vi "CLASS - Generate2DTest.vi"(8 "error in (no error)":errorcluster, 11 "Local":T6) -> (0 "error out":errorcluster, 3 "Local Out":T6)   [LabVIEW 2020]
doc: "Generate the 2D graph"
uses:
  Controls/2DParameters.ctl
  _Controls/Datas.ctl
  _Controls/PointPropertyMultipleLabel.ctl
  _Controls/Style.ctl
  _Controls/2DData.ctl
types:
  T1 = typedef "2DParameters.ctl" = cluster{"Plot":refnum<vi>, "Data":T2, "Display":cluster{"Choice":enum16{"All", "Train", "Test"}, "Indexe":cluster{"X":i32, "Y":i32}}, "Property":T3}
  T2 = typedef "Datas.ctl" = cluster{"Split":cluster{"X Train":dbl[][], "X Test":dbl[][], "Y Train":dbl[][], "Y Test":dbl[][]}, "Predict":dbl[][]}
  T3 = typedef "PointPropertyMultipleLabel.ctl" = cluster{"Train Style":T4, "Test OK Style":T4, "Label Color":u32[], "Test NO OK":cluster{"Style":T4, "Color":u32}}
  T4 = typedef "Style.ctl" = enum16{"Empty circle", "Full circle", "Empty square", "Full square", "Cross"}
  T5 = typedef "2DData.ctl" = cluster{"Tag":i32, "X":dbl[], "Y":dbl[]}
  T6 = cluster{"Parameters":T1, "2D Array":cluster{"X":dbl[], "Y":dbl[]}[], "Rating 2D Array":T5[], "Point ID":cluster{"DataUse":enum16{"Dataset", "Train", "Test"}, "Color":u32}[], "GoodPredict":i32}
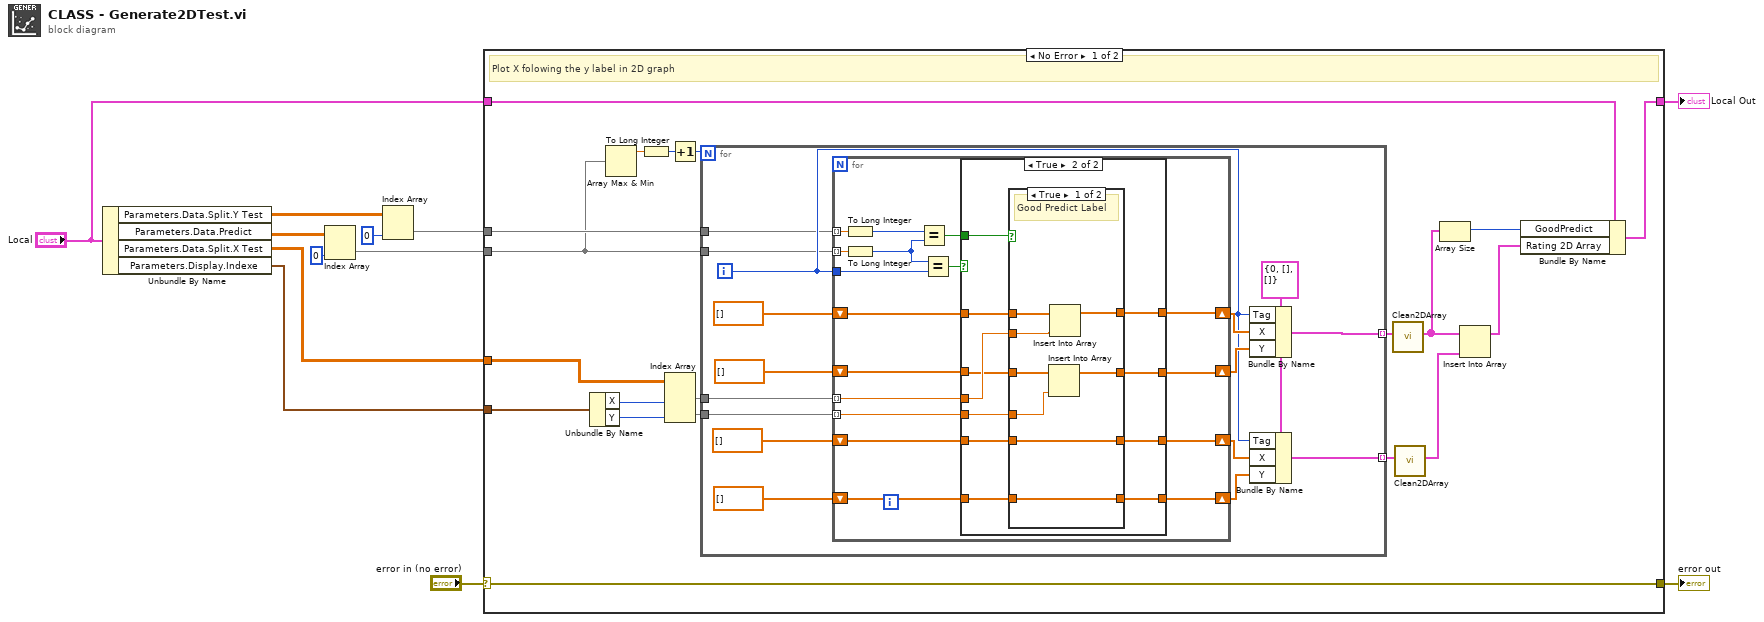
[diagram p0: block diagram]
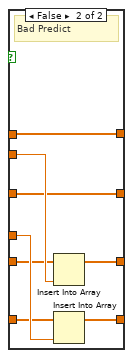
[diagram p3: hidden frame]
diagram:
  n1 = Unbundle By Name("Local") -> ("Parameters.Data.Split.Y Test"=w8:dbl[][], "Parameters.Data.Predict"=w9:dbl[][], "Parameters.Data.Split.X Test"=w5:dbl[][], "Parameters.Display.Indexe"=w2:cluster{"X":i32, "Y":i32})
  n2 = Index Array(array=w9, index (col)=0 ("disabled index (col)")) -> (element=w6:dbl[])  [unwired: 1 in]
  n3 = Index Array(array=w8, index (col)=0 ("disabled index (col)")) -> (element=w7:dbl[])  [unwired: 1 in]
  n4 = case shown="No Error" "error in (no error)" {
    selector: "error in (no error)" -> [w17 w98]
    tunnel: w5 -> [w27 _]
    tunnel: w6 -> [w20 _]
    tunnel: [w17 w98] -> w12
    tunnel: w7 -> [w21 _]
    tunnel: "Local" -> [w24 w97]
    tunnel: [w23 w97] -> w3
    tunnel: w2 -> [w19 _]
    frame No Error {
      # "Plot X folowing the y label in 2D graph"
      n5 = Unbundle By Name(w19) -> ("X"=w26:i32, "Y"=w25:i32)
      n6 = Array Max & Min(array=w20) -> (max value=w30:dbl)  [unwired: 3 out]
      n7 = To Long Integer(number=w30) -> (32bit integer=w29:i32)
      n8 = Index Array(array=w27, index (col) #1=w26, index (col) #2=w25) -> (element #1=w32:dbl[], element #2=w31:dbl[])  [unwired: 2 in]
      n9 = Increment(x=w29) -> (x+1=w28:i32)
      n10 = for {
        N: w28 -> [_]
        tunnel: w32 -> [w36]
        tunnel: w31 -> [w48]
        tunnel: w20 -> [w34]
        tunnel: [w45] -> w16 mode=indexing
        tunnel: w21 -> [w35]
        tunnel: [w40] -> w14 mode=indexing
        i -> [w37]
        w33 = T5 {"Tag"=0, "X"=[], "Y"=[]} ("2D Data")
        n11 = for {
          tunnel: w34 -> [w65] mode=indexing
          tunnel: w36 -> [w64] mode=indexing
          tunnel: w48 -> [w63] mode=indexing
          shift-right: [w61] -> w47
          shift-left: dbl[] [] -> [w60]
          shift-right: [w62] -> w46
          shift-left: dbl[] [] -> [w59]
          tunnel: w37 -> [w58]
          tunnel: w35 -> [w56] mode=indexing
          shift-right: [w49] -> w38
          shift-left: dbl[] [] -> [w51]
          shift-right: [w50] -> w39
          shift-left: dbl[] [] -> [w52]
          n12 = To Long Integer(number=w56) -> (32bit integer=w55:i32)
          n13 = To Long Integer(number=w65) -> (32bit integer=w53:i32)
          n14 = Equal?(x=w55, y=w53) -> (x = y?=w54:bool)
          n15 = Equal?(x=w53, y=w58) -> (x = y?=w57:bool)
          n16 = case shown="True" w57 {
            tunnel: w64 -> [_ w79]
            tunnel: w63 -> [_ w75]
            tunnel: [w68 w77] -> w62
            tunnel: [w69 w78] -> w61
            tunnel: w60 -> [w69 w80]
            tunnel: w59 -> [w68 w76]
            tunnel: w54 -> [_ w74]
            tunnel: w51 -> [w66 w71]
            tunnel: w52 -> [w67 w73]
            tunnel: [w67 w72] -> w50
            tunnel: [w66 w70] -> w49
            frame False {
            }
            frame True {
              n17 = case shown="True" w74 {
                tunnel: w80 -> [w88 w90]
                tunnel: w79 -> [w87 w96]
                tunnel: [w86 w90] -> w78
                tunnel: [w85 w91] -> w77
                tunnel: w76 -> [w84 w91]
                tunnel: w75 -> [w83 w95]
                tunnel: w73 -> [w81 w94]
                tunnel: [w81 w89] -> w72
                tunnel: w71 -> [w82 w93]
                tunnel: [w82 w92] -> w70
                frame True {
                  # "Good Predict Label"
                  n18 = Insert Into Array(array=w84, new element=w83) -> (w85:dbl[])  [unwired: 1 in]
                  n19 = Insert Into Array(array=w88, new element=w87) -> (w86:dbl[])  [unwired: 1 in]
                }
                frame False {
                  # "Bad Predict"
                  n20 = Insert Into Array(array=w93, new element=w96) -> (w92:dbl[])  [unwired: 1 in]
                  n21 = Insert Into Array(array=w94, new element=w95) -> (w89:dbl[])  [unwired: 1 in]
                }
              }
            }
          }
        }
        n22 = Bundle By Name(cluster=w33, "Tag"=w37, "X"=w47, "Y"=w46) -> (w45:T5)
        n23 = Bundle By Name(cluster=w33, "Tag"=w37, "X"=w38, "Y"=w39) -> (w40:T5)
      }
      n24 = call "Clean2DArray.vi"("Array2D"=w16) -> ("Array2DClean"=w15:T5[])  [unwired: 10 in]
      n25 = call "Clean2DArray.vi"("Array2D"=w14) -> ("Array2DClean"=w13:T5[])  [unwired: 10 in]
      n26 = Array Size(array=w15) -> (size(s)=w22:i32)
      n27 = Insert Into Array(array=w15, new element=w13) -> (w18:T5[])  [unwired: 1 in]
      n28 = Bundle By Name(cluster=w24, "GoodPredict"=w22, "Rating 2D Array"=w18) -> (w23:T6)
    }
    frame Error {
    }
  }
  "error out" <- w12
  "Local Out" <- w3
